vi "PWM_SetValue.vi"(5 "PWM":T1=1 items=["Invalid"=0, "PWM1"=1, "PWM2"=2, "PWM9"=9, "PWM10"=10], 7 "High (uSec)":u32, 9 "Period (uSec)":u32, 11 "error in":errorcluster) -> (15 "error out":errorcluster)   [LabVIEW 2009, in "PWM.lvlib"]
doc: "This function will feed the FPGA with a digital signal that the FPGA then will continuously feed to the Side car, for as long as it is enabled. The function requires a correct input port in the form of a PWM_Name (see the CTL file). It also require how long the signal should be high in uSec and how long each period should be. This will then construct an acceptable PWM signal."
uses:
  PWM.lvlib
  PWM_Name.ctl
  <vilib>/rvi/interface/nirviReadWriteControl/nirviReadWriteControl.xnode
  FPGA Bitfiles/scmproject.lvproj_FPGA Target_RobotFPGA.vi.lvbitx
  RobotFPGA.vi
  <vilib>/LabVIEW Targets/FPGA/Rio/nirio_HostInterface/nirio_WriteBig.vi
  <vilib>/rvi/errors/niLvFpgaAdjustHostInterfaceError.vi
  <vilib>/rvi/interface/common/niFpgaNodeNameForErrorReporting.ctl
  <vilib>/rvi/errors/niLvFpgaWhatHappensToTopLevelVI.ctl
  FPGA.lvlib
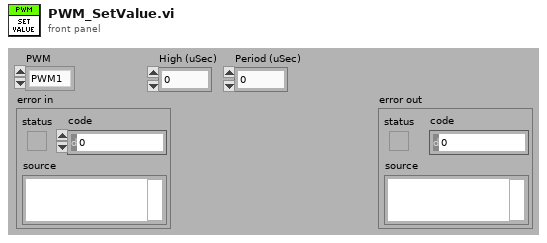
[diagram p1: front panel]
types:
  T1 = typedef "PWM.lvlib/PWM_Name.ctl" = u16
  T2 = typedef "niFpgaNodeNameForErrorReporting.ctl" = enum16{"Open FPGA VI Reference", "Read/Write Control", "Invoke Method: Abort", "Invoke Method: Acknowledge IRQ", "Invoke Method: Download", "Invoke Method: FIFO.Configure", "Invoke Method: FIFO.Read", "Invoke Method: FIFO.Start", "Invoke Method: FIFO.Stop", "Invoke Method: FIFO.Write", "Invoke Method: Reset", "Invoke Method: Run", "Invoke Method: Wait on IRQ", "Close FPGA VI Reference"}
  T3 = typedef "niLvFpgaWhatHappensToTopLevelVI.ctl" = enum16{"top level VI scripted behind XNode", "top level VI inlined behind XNode"}
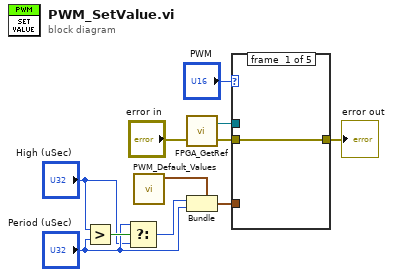
[diagram p0: block diagram]
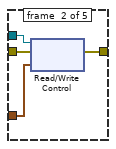
[diagram p2: hidden frame]
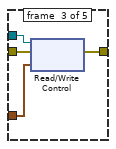
[diagram p3: hidden frame]
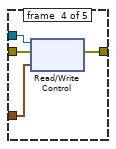
[diagram p4: hidden frame]
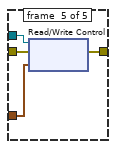
[diagram p5: hidden frame]
diagram:
  n1 = Greater?(x="High (uSec)", y="Period (uSec)") -> (0:w7:bool)
  n2 = Select(t="Period (uSec)", s=w7, f="High (uSec)") -> (s? t:f=w8:u32)
  n3 = call "PWM_Default_Values.vi"() -> ("PWM_default"=w9:cluster{"High (uSec)":u32, "Period (uSec)":u32})  [unwired: 11 in]
  n4 = call "FPGA_GetRef.vi"("error in (no error)"="error in") -> ("error out"=w2:errorcluster, "FPGA_Ref"=w1:refnum<k20>)  [unwired: 1 in]
  n5 = Bundle(cluster=w9, "High (uSec)"=w8, "Period (uSec)"="Period (uSec)") -> (w10:cluster{"High (uSec)":u32, "Period (uSec)":u32})
  n6 = case shown="9" "PWM" {
    tunnel: w1 -> [_ w13 w44 w75 w106]
    tunnel: w2 -> [w12 w16 w47 w78 w109]
    tunnel: [w12 w15 w46 w77 w108] -> w4
    tunnel: w10 -> [_ w14 w45 w76 w107]
    frame #0 {
    }
    frame #1 {
      n7 = xnode "Read/Write Control"("FPGA VI Reference In"=w13, "error in"=w16, "PWM1"=w14) -> ("error out"=w15:errorcluster)  [unwired: 1 out]
    }
    frame #2 {
      n8 = xnode "Read/Write Control"("FPGA VI Reference In"=w44, "error in"=w47, "PWM2"=w45) -> ("error out"=w46:errorcluster)  [unwired: 1 out]
    }
    frame #3 {
      n9 = xnode "Read/Write Control"("FPGA VI Reference In"=w75, "error in"=w78, "PWM9"=w76) -> ("error out"=w77:errorcluster)  [unwired: 1 out]
    }
    frame #4 {
      n10 = xnode "Read/Write Control"("FPGA VI Reference In"=w106, "error in"=w109, "PWM10"=w107) -> ("error out"=w108:errorcluster)  [unwired: 1 out]
    }
  }
  "error out" <- w4
